vi "Measure [MSR] Core.vi"(8 "error in (no error)":errorcluster, 9 "measurement type (voltage)":i32(ring)=1 items=["Voltage"=1, "Current"=0], 10 "channel name (\"CHANNEL1\")":string="CHANNEL1", 11 "Cs++DCPwr in":refnum<class "CS++DCPwr.lvclass">) -> (0 "error out":errorcluster, 2 "measurement":dbl format="%^.2e", 3 "CS++DCPwr out":refnum<class "CS++DCPwr.lvclass">)   [LabVIEW 2013, in "CS++DCPwr.lvlib" / "CS++DCPwr.lvclass"]
doc: "This VI takes a single measurement on the channel you specify.\n\nNotes:\n\n(1) This VI is part of the IviDCPwrMeasure [MSR] extension group."
uses:
  CS++DCPwr.lvclass
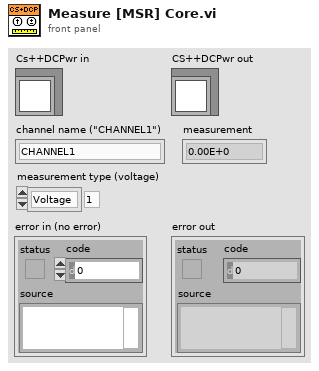
[diagram p1: front panel]
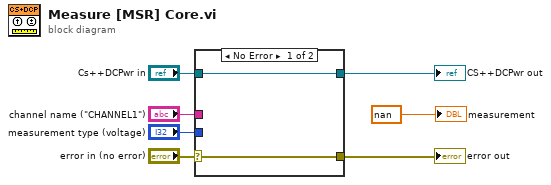
[diagram p0: block diagram]
diagram:
  n1 = case shown="No Error" "error in (no error)" {
    selector: "error in (no error)" -> [w8 w11]
    tunnel: [w8 w11] -> w6
    tunnel: [w9 w10] -> w4
    tunnel: "Cs++DCPwr in" -> [w9 w10]
    tunnel: "channel name (\"CHANNEL1\")" -> [_ _]
    tunnel: "measurement type (voltage)" -> [_ _]
    frame No Error {
    }
    frame Error {
    }
  }
  "error out" <- w6
  "CS++DCPwr out" <- w4
  "measurement" <- nan ("measurement")
